vi "Update Last VI List to Menu.vi"(0 "LastVIs":string[](array[string]), 1 "menu reference":refnum<k9>, 11 "error in (no error)":errorcluster) -> (15 "error out":errorcluster)   [LabVIEW 2014]
doc: "Updates the recent used VIs list in the RTM."
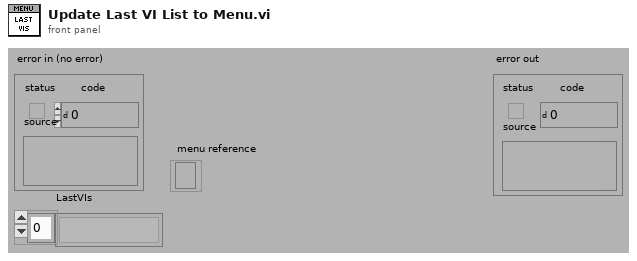
[diagram p1: front panel]
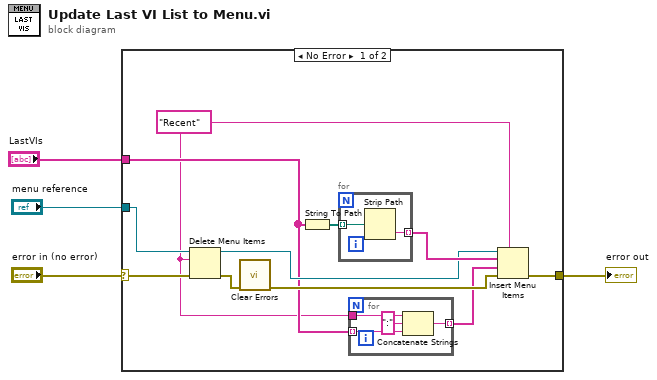
[diagram p0: block diagram]
diagram:
  n1 = case shown="No Error" "error in (no error)" {
    selector: "error in (no error)" -> [w13 w22]
    tunnel: [w11 w22] -> w3
    tunnel: "menu reference" -> [w12 _]
    tunnel: "LastVIs" -> [w7 _]
    frame No Error {
      w6 = "Recent" ("menu tag")
      n2 = Delete Menu Items(6:w13, 8:w6, 9:w12) -> (0:w9:errorcluster, 3:w10:refnum<k9>)  [unwired: 1 in]
      n3 = call <vilib>:"Clear Errors.vi"("error in (no error)"=w9) -> ("error out"=w8:errorcluster)  [unwired: 5 in, 1 out]
      n4 = String To Path(string=w7) -> (path=w14:path[])
      n5 = for {
        tunnel: w14 -> [w21] mode=indexing
        tunnel: [w20] -> w15 mode=indexing
        n6 = Strip Path(path=w21) -> (name=w20:string)  [unwired: 1 out]
      }
      n7 = for {
        tunnel: w7 -> [w18] mode=indexing
        tunnel: w6 -> [w17]
        tunnel: [w16] -> w5 mode=indexing
        n8 = Concatenate Strings(w17, ":" ("string"), w18) -> (w16:string)
      }
      n9 = Insert Menu Items(5:w6, 6:w8, 7:w5, 8:w15, 9:w10) -> (0:w11:errorcluster)  [unwired: 1 in, 2 out]
    }
    frame Error {
    }
  }
  "error out" <- w3
